vi "DispenserTesting.vi"() -> ()   [LabVIEW 2019]
uses:
  Other Models/EFD Ultimus V/EFD Ultimus V.lvlib
panel:
  out "Ultimus V Feedback Data":string
  out "Iterations":i32
  in  "milliseconds to wait":u32=2000
  in  "Stop Button":bool
  in  "Command Code":string="G91"
  out "error out":errorcluster
  in  "Serial Configuration":T1={"Baud Rate "=115200, "Parity "=0, "Data Bits "=8, "Stop Bits"=10} {"Stop Bits" items=["1.0"=10, "1.5"=15, "2.0"=20]; "Data Bits" items=["7"=7, "8"=8]; "Parity" items=["None", "Odd", "Even"]; "Baud Rate" items=["9600"=9600, "19200"=19200, "38400"=38400, "115200"=115200]}
  in  "VISA resource name":refnum<visa-resource-name>="COM5"
  in  "PressureSet":dbl=30.0
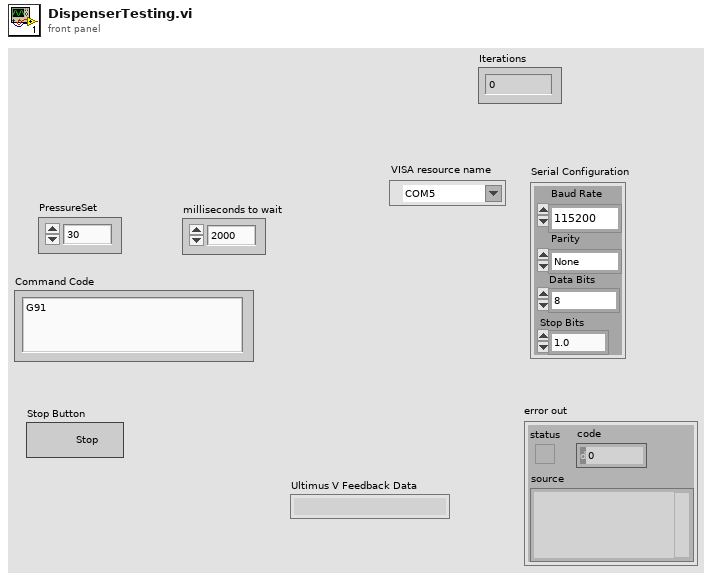
[diagram p1: front panel]
types:
  T1 = cluster{"Baud Rate ":u32, "Parity ":u16, "Data Bits ":u16, "Stop Bits":u16}
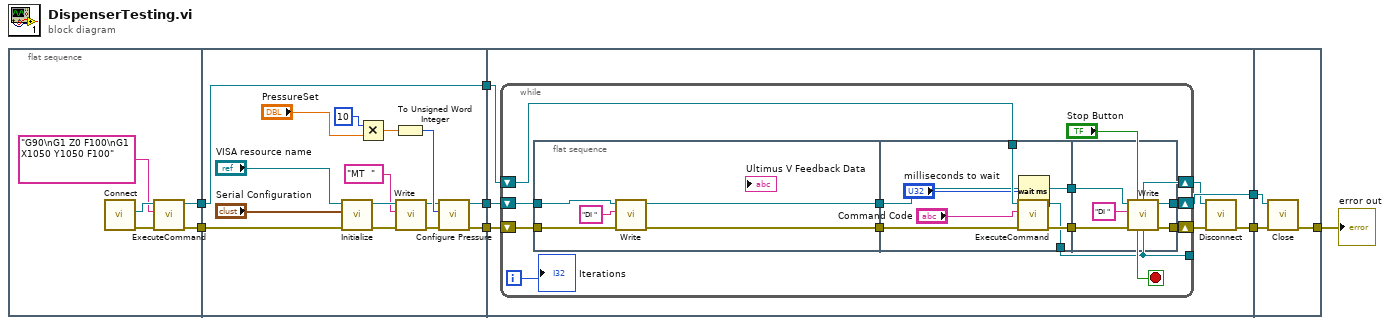
[diagram p0: block diagram]
diagram:
  n1 = flat-sequence {
    tunnel: [w10] -> w2
    tunnel: [w9] -> w1
    tunnel: [w16] -> w7
    tunnel: [w17] -> w6
    tunnel: [w15] -> w3
    tunnel: w2 -> [w15]
    tunnel: w1 -> [w14]
    tunnel: w7 -> [w35]
    tunnel: w6 -> [w34]
    tunnel: [w29] -> w5
    tunnel: [w33] -> w4
    tunnel: w3 -> [w32]
    tunnel: w5 -> [w67]
    tunnel: w4 -> [w66]
    tunnel: [w65] -> w8
    frame #0 {
      n2 = call "Connect.vi"() -> ("error out"=w12:errorcluster, "controller"=w13:refnum<k24>)  [unwired: 10 in]
      n3 = call "ExecuteCommand.vi"("error in (no error)"=w12, "Command Code"="G90\nG1 Z0 F100\nG1 X1050 Y1050 F100", "controller in"=w13) -> ("error out"=w9:errorcluster, "controller out"=w10:refnum<k24>)  [unwired: 6 in, 1 out]
    }
    frame #1 {
      n4 = call "Initialize.vi"("error in (no error)"=w14, "Serial Configuration"="Serial Configuration", "VISA resource name"="VISA resource name") -> ("error out"=w23:errorcluster, "VISA resource name out"=w22:refnum<visa-resource-name>)  [unwired: 7 in]
      n5 = Multiply(x=10, y="PressureSet") -> (x*y=w25:dbl)
      n6 = To Unsigned Word Integer(number=w25) -> (unsigned 16bit integer=w26:u16)
      n7 = call "Write.vi"("error in (no error)"=w23, "Command To Write"="MT  ", "VISA resource name"=w22) -> ("error out"=w27:errorcluster, "VISA resource name out"=w24:refnum<visa-resource-name>)  [unwired: 7 in]
      n8 = call "Configure Pressure.vi"("error in (no error)"=w27, "Pressure Setting (0000)"=w26, "VISA resource name"=w24) -> ("error out"=w17:errorcluster, "VISA resource name out"=w16:refnum<visa-resource-name>)  [unwired: 7 in]
    }
    frame #2 {
      n9 = while {
        shift-right: [w43] -> w33
        shift-left: w35 -> [w45]
        shift-right: [w44] -> w30
        shift-left: w34 -> [w46]
        tunnel: [w37] -> _
        shift-right: [w37] -> w31
        shift-left: w32 -> [w47]
        i -> [w36]
        stop <- "Stop Button" stop-if-true
        n10 = flat-sequence {
          tunnel: w46 -> [w52]
          tunnel: w45 -> [w50]
          tunnel: [w49] -> w41
          tunnel: [w48] -> w40
          tunnel: w47 -> [w59]
          tunnel: [w58] -> w42
          tunnel: w41 -> [w58]
          tunnel: w40 -> [w57]
          tunnel: [w55] -> w39
          tunnel: [w54] -> w37
          tunnel: [w63] -> w44
          tunnel: [w62] -> w43
          tunnel: w42 -> [w61]
          tunnel: w39 -> [w60]
          frame #0 {
            n11 = call "Write.vi"("error in (no error)"=w52, "Command To Write"="DI ", "VISA resource name"=w50) -> ("error out"=w48:errorcluster, "VISA resource name out"=w49:refnum<visa-resource-name>)  [unwired: 7 in]
          }
          frame #1 {
            n12 = call "ExecuteCommand.vi"("error in (no error)"=w57, "Command Code"="Command Code", "controller in"=w59) -> ("error out"=w55:errorcluster, "controller out"=w54:refnum<k24>)  [unwired: 6 in, 1 out]
            n13 = Wait (ms)(milliseconds to wait="milliseconds to wait") -> ()  [unwired: 1 out]
          }
          frame #2 {
            n14 = call "Write.vi"("error in (no error)"=w60, "Command To Write"="DI ", "VISA resource name"=w61) -> ("error out"=w63:errorcluster, "VISA resource name out"=w62:refnum<visa-resource-name>)  [unwired: 7 in]
          }
        }
        "Iterations" <- w36
      }
      n15 = call "Disconnect.vi"("error in (no error)"=w30, "controller"=w31) -> ("error out"=w29:errorcluster)  [unwired: 9 in]
    }
    frame #3 {
      n16 = call "Close.vi"("error in (no error)"=w67, "VISA resource name"=w66) -> ("error out"=w65:errorcluster)  [unwired: 9 in]
    }
  }
  "error out" <- w8
